vi "CileckItem(Event Callback).vi"(4 "Mgessage":refnum<user-event>, 5 "Event Data":cluster{"sender":refnum<k24>, "e":refnum<k24>}, 6 "Control Ref":refnum<k24>, 7 "Event Common Data":T1) -> ()   [LabVIEW 2019]
uses:
  System.Windows.Forms
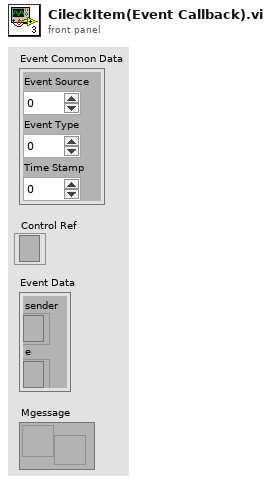
[diagram p1: front panel]
types:
  T1 = cluster{"Event Source":i32, "Event Type":u32, "Time Stamp":u32}
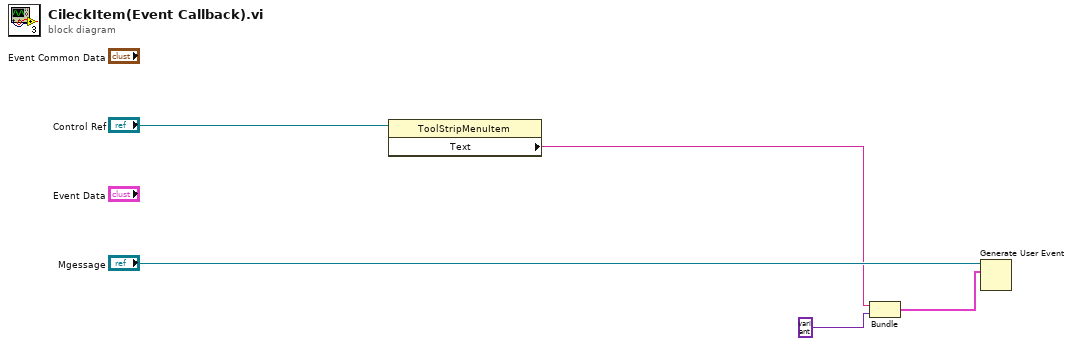
[diagram p0: block diagram]
diagram:
  n1 = property class="ToolStripMenuItem"(reference="Control Ref") -> ("Text"=w2:string)  [unwired: 1 in, 2 out]
  n2 = Bundle("Text"=w2, "Value"=variant) -> (w1:cluster{"Text":string, "Value":variant})  [unwired: 1 in]
  n3 = Generate User Event(user event="Mgessage", event data cluster=w1) -> ()  [unwired: 2 in, 2 out]
